vi "get time stamp.vi"(8 "error in (no error)":errorcluster, 11 "Log File in":refnum<class "Events Log File.lvclass">) -> (0 "error out":errorcluster, 2 "time stamp":string, 3 "Log File out":refnum<class "Events Log File.lvclass">)   [LabVIEW 2018, in "Events Log File.lvclass"]
uses:
  Events Log File.lvclass
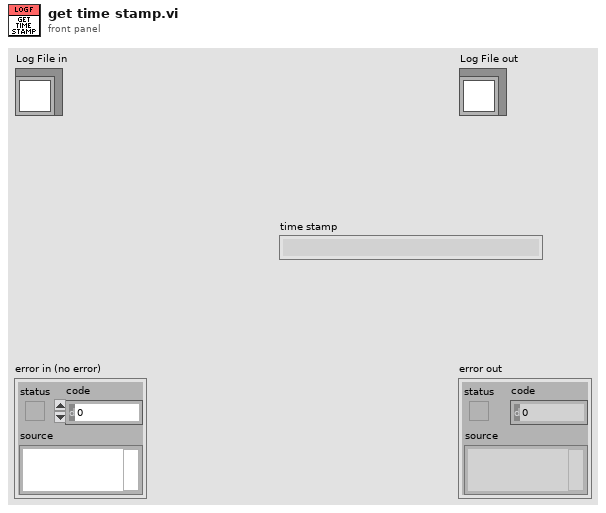
[diagram p1: front panel]
types:
  T1 = typedef "LVDateTimeRec.ctl" = cluster{"fractional second":dbl, "second":i32, "minute":i32, "hour":i32, "day of month":i32, "month":i32, "year":i32, "day of week":i32, "day of year":i32, "DST":i32}
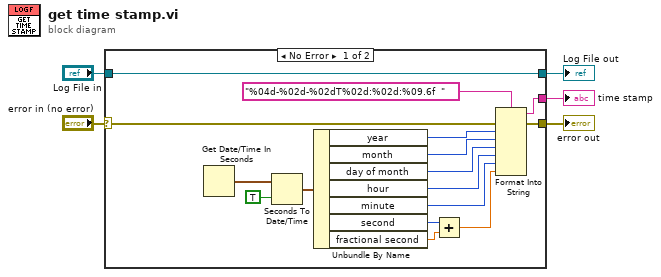
[diagram p0: block diagram]
diagram:
  n1 = case shown="No Error" "error in (no error)" {
    selector: "error in (no error)" -> [w10 w23]
    tunnel: [w8 w23] -> w4
    tunnel: [w18 w22] -> w2
    tunnel: "Log File in" -> [w18 w22]
    tunnel: [w9 _] -> w1
    frame No Error {
      n2 = Get Date/Time In Seconds() -> (seconds since 1Jan1904=w7:timestamp)
      n3 = Seconds To Date/Time(time stamp (now)=w7, to UTC (F)=TRUE) -> (date time rec=w21:T1)
      n4 = Unbundle By Name(w21) -> ("year"=w17:i32, "month"=w16:i32, "day of month"=w15:i32, "hour"=w14:i32, "minute"=w13:i32, "second"=w20:i32, "fractional second"=w19:dbl)
      n5 = Add(x=w20, y=w19) -> (x+y=w12:dbl)
      n6 = Format Into String(format string="%04d-%02d-%02dT%02d:%02d:%09.6f  ", error in=w10, w17, w16, w15, w14, w13, w12) -> (resulting string=w9:string, error out=w8:errorcluster)  [unwired: 1 in]
    }
    frame Error {
    }
  }
  "error out" <- w4
  "Log File out" <- w2
  "time stamp" <- w1
